vi "menuBuilder.vi"(8 "error in (no error)":errorcluster, 11 "Menu in":refnum<k9>) -> (0 "error out":errorcluster)   [LabVIEW 2015]
doc: "Builds menu for main front panel.\nTo be used on \"Tausand AB1000 Acquisition Example.vi\"."
uses:
  <vilib>/Utility/miscctls.llb/LVMenuShortCut.ctl
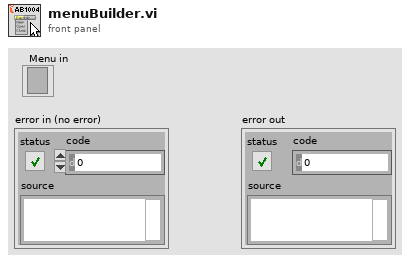
[diagram p1: front panel]
types:
  T1 = typedef "LVMenuShortCut.ctl" = cluster{"Include Shift Key?":bool, "Include Ctrl Key?":bool, "Shortcut Key":string}
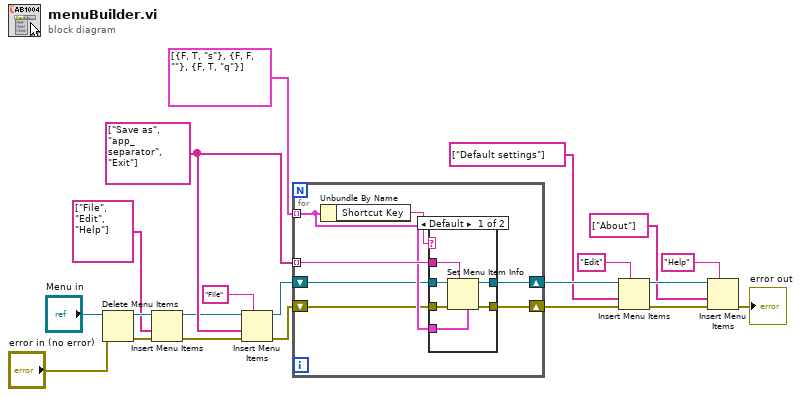
[diagram p0: block diagram]
diagram:
  w16 = string[] ["Save as", "app_separator", "Exit"] ("item tags")
  n1 = Delete Menu Items(6:"error in (no error)", 9:"Menu in") -> (0:w15:errorcluster, 3:w14:refnum<k9>)  [unwired: 2 in]
  n2 = Insert Menu Items(6:w15, 7:string[] ["File", "Edit", "Help"] ("item tags"), 9:w14) -> (0:w3:errorcluster, 3:w4:refnum<k9>)  [unwired: 3 in, 1 out]
  n3 = Insert Menu Items(5:"File" ("menu tag"), 6:w3, 7:w16, 9:w4) -> (0:w19:errorcluster, 3:w18:refnum<k9>)  [unwired: 2 in, 1 out]
  n4 = for {
    tunnel: w16 -> [w28] mode=indexing
    tunnel: T1[] [{"Include Shift Key?"=FALSE, "Include Ctrl Key?"=TRUE, "Shortcut Key"="s"}, {"Include Shift Key?"=FALSE, "Include Ctrl Key?"=FALSE, "Shortcut Key"=""}, {"Include Shift Key?"=FALSE, "Include Ctrl Key?"=TRUE, "Shortcut Key"="q"}] -> [w26] mode=indexing
    shift-right: [w23] -> w20
    shift-left: w19 -> [w24]
    shift-right: [w22] -> w21
    shift-left: w18 -> [w25]
    n5 = Unbundle By Name(w26) -> ("Shortcut Key"=w27:string)
    n6 = case shown="Default" w27 {
      tunnel: w28 -> [w34 _]
      tunnel: w26 -> [w33 _]
      tunnel: w25 -> [w32 w36]
      tunnel: w24 -> [w31 w35]
      tunnel: [w30 w35] -> w23
      tunnel: [w29 w36] -> w22
      frame Default {
        n7 = Set Menu Item Info(4:w33, 7:w34, 8:w31, 11:w32) -> (0:w30:errorcluster, 3:w29:refnum<k9>)  [unwired: 3 in]
      }
      frame "" {
      }
    }
  }
  n8 = Insert Menu Items(5:"Edit" ("menu tag"), 6:w20, 7:string[] ["Default settings"] ("item tags"), 9:w21) -> (0:w10:errorcluster, 3:w11:refnum<k9>)  [unwired: 2 in, 1 out]
  n9 = Insert Menu Items(5:"Help" ("menu tag"), 6:w10, 7:string[] ["About"] ("item tags"), 9:w11) -> (0:→"error out":errorcluster)  [unwired: 2 in, 2 out]
